vi "Reference Image Path.vi"(7 "Get/Set":enum16{"Get", "Set"}(ring), 8 "error in (no error)":errorcluster, 9 "Image Path":path, 10 "Image ID/Path":string, 11 "FlexWorktable in":refnum<class "FlexWorktable.lvclass">) -> (0 "error out":errorcluster, 1 "Image Path":path, 3 "FlexWorktable out":refnum<class "FlexWorktable.lvclass">)   [LabVIEW 2024, in "FlexWorktable.lvclass"]
uses:
  FlexWorktable.lvclass
  FlexWorktable.lvclass/FlexWorktable.ctl
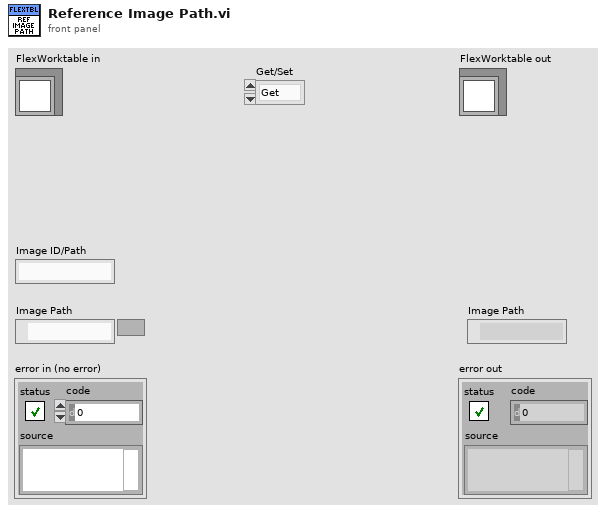
[diagram p1: front panel]
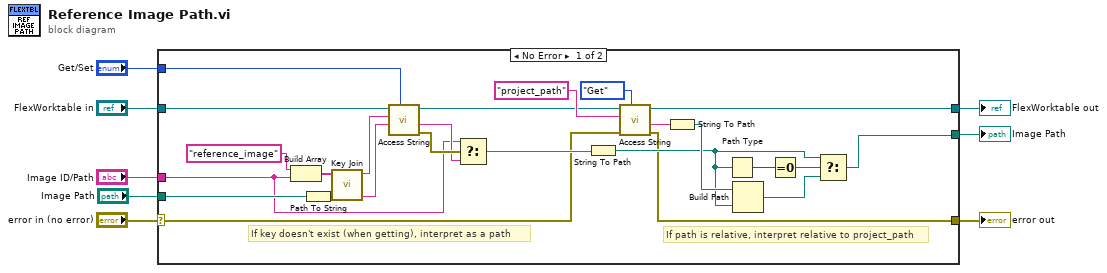
[diagram p0: block diagram]
diagram:
  n1 = case shown="No Error" "error in (no error)" {
    selector: "error in (no error)" -> [w9 w34]
    tunnel: [w16 w34] -> w7
    tunnel: [w14 w33] -> w5
    tunnel: "FlexWorktable in" -> [w19 w33]
    tunnel: "Get/Set" -> [w32 _]
    tunnel: "Image ID/Path" -> [w11 _]
    tunnel: "Image Path" -> [w20 _]
    tunnel: [w17 _] -> w1
    frame No Error {
      # "If key doesn't exist (when getting), interpret as a path"
      # "If path is relative, interpret relative to project_path"
      n2 = Build Array("reference_image" ("element"), w11) -> (w31:string[])
      n3 = Path To String(path=w20) -> (string=w28:string)
      n4 = call "Key Join.vi"("Key Elements"=w31) -> ("Key"=w30:string)  [unwired: 10 in]
      n5 = call-dynamic "Access String.vi"("Get/Set"=w32, "Value in"=w28, "Key"=w30, "FlexWorktable in"=w19) -> ("error out"=w13:errorcluster, "Value out"=w12:string, "FlexWorktable out"=w15:refnum<class "FlexWorktable.lvclass">)  [unwired: 5 in]
      n6 = Select(t=w11, s=w13, f=w12) -> (s? t:f=w10:string)
      n7 = String To Path(string=w10) -> (path=w18:path)
      n8 = call-dynamic "Access String.vi"("Get/Set"=enum16{"Get", "Set"}."Get", "error in (no error)"=w9, "Key"="project_path", "FlexWorktable in"=w15) -> ("error out"=w16:errorcluster, "Value out"=w25:string, "FlexWorktable out"=w14:refnum<class "FlexWorktable.lvclass">)  [unwired: 5 in]
      n9 = String To Path(string=w25) -> (path=w24:path)
      n10 = Path Type(1:w18) -> (0:w23:i16)
      n11 = Build Path(base path=w24, name or relative path=w18) -> (appended path=w21:path)
      n12 = Equal To 0?(x=w23) -> (x = 0?=w22:bool)
      n13 = Select(t=w18, s=w22, f=w21) -> (s? t:f=w17:path)
    }
    frame Error {
    }
  }
  "error out" <- w7
  "FlexWorktable out" <- w5
  "Image Path" <- w1
